vi "ELVIS III v1.0 Shutdown PWM.vi"(8 "error in (no error)":errorcluster, 10 "Channel":T1, 11 "myRIO Ref In":T2) -> (0 "error out":errorcluster, 3 "myRIO Ref Out":T2)   [LabVIEW 2021]
uses:
  <vilib>/myRIO/Common/Instrument Driver Framework/Utilities/typedefs/myRIO v1.0 Reference.ctl
  <vilib>/myRIO/Common/Instrument Driver Framework/Utilities/typedefs/Generic FPGA Reference.ctl
  <vilib>/myRIO/Common/Instrument Driver Framework/myRIO v1.0/PWM/typedefs/PWM Channels Enum.ctl
  <vilib>/myRIO/Common/Instrument Driver Framework/ELVIS III v1.0/PWM/typedefs/ELVIS III PWM Channels FPGA Reference.ctl
  <vilib>/rvi/errors/niLvFpgaAdjustHostInterfaceError.vi
  <vilib>/rvi/interface/nirviReadWriteControl/nirviReadWriteControl.xnode
  NiFpgaLv.dll
  <vilib>/rvi/interface/Simulation/niFpgaSimulationCallBeginRW.vi
panel:
  # "This VI turns off the specified PWM channel and zeroes out all of its registers."
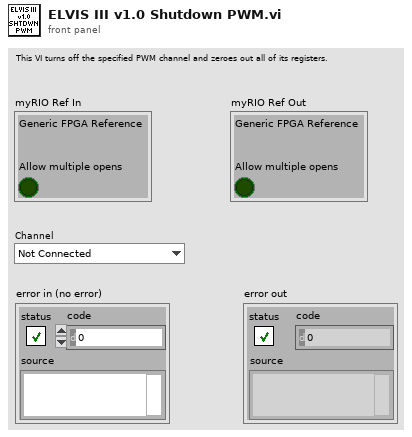
[diagram p1: front panel]
types:
  T1 = typedef "PWM Channels Enum.ctl" = enum16{"Not Connected", "C/PWM0", "C/PWM1", "A/PWM0", "A/PWM1", "A/PWM2", "A/PWM3", "A/PWM4", "A/PWM5", "A/PWM6", "A/PWM7", "A/PWM8", "A/PWM9", "A/PWM10", "A/PWM11", "A/PWM12", "A/PWM13", "A/PWM14", "A/PWM15", "A/PWM16", "A/PWM17", "A/PWM18", "A/PWM19", "B/PWM0", "B/PWM1", "B/PWM2", "B/PWM3", "B/PWM4", "B/PWM5", "B/PWM6", "B/PWM7", "B/PWM8", "B/PWM9", "B/PWM10", "B/PWM11", "B/PWM12", "B/PWM13", "B/PWM14", "B/PWM15", "B/PWM16", "B/PWM17", "B/PWM18", "B/PWM19", "PWM/PWM0", "PWM/PWM1", "PWM/PWM2", "PWM/PWM3", "PWM/PWM4", "PWM/PWM5", "PWM/PWM6", "PWM/PWM7", "PWM/PWM8", "PWM/PWM9"}
  T2 = typedef "myRIO v1.0 Reference.ctl" = cluster{"Generic FPGA Reference":T3, "Allow multiple opens":bool}
  T3 = typedef "Generic FPGA Reference.ctl" = refnum<k20>
  T4 = typedef "ELVIS III PWM Channels FPGA Reference.ctl" = refnum<k20>
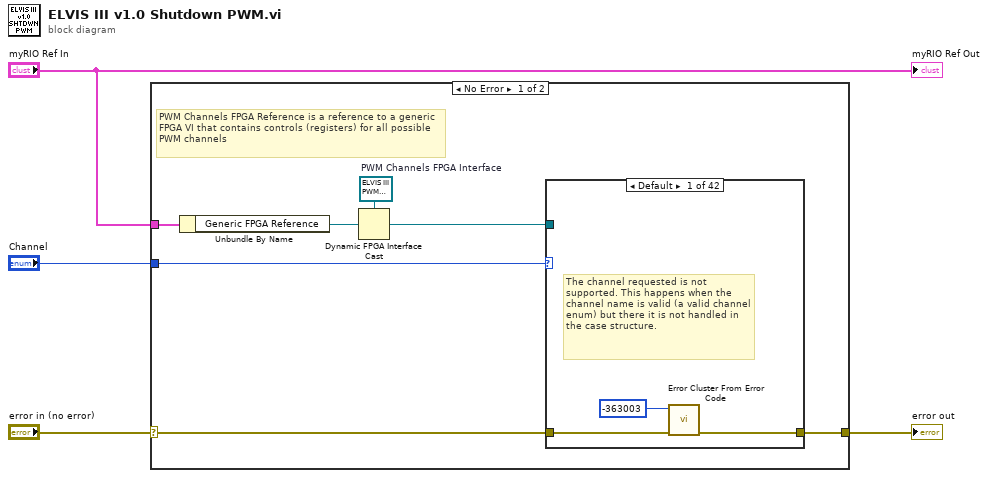
[diagram p0: block diagram]
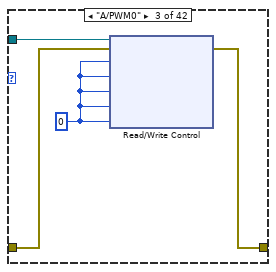
[diagram p3: hidden frame]
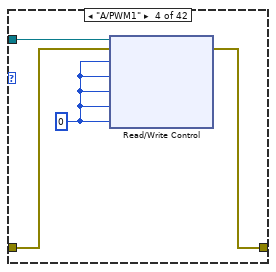
[diagram p4: hidden frame]
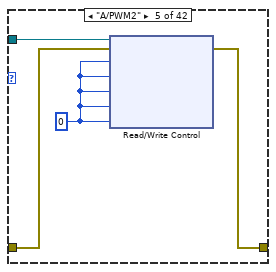
[diagram p5: hidden frame]
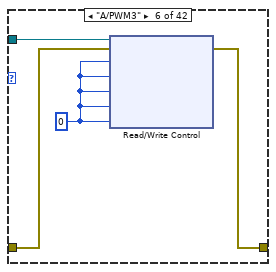
[diagram p6: hidden frame]
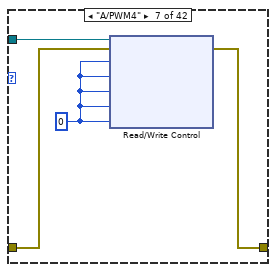
[diagram p7: hidden frame]
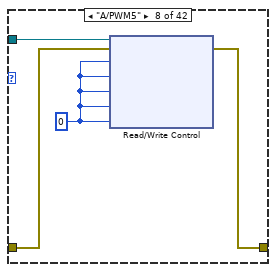
[diagram p8: hidden frame]
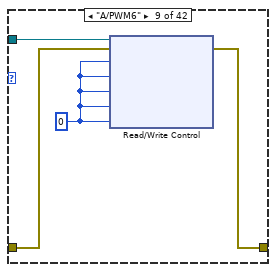
[diagram p9: hidden frame]
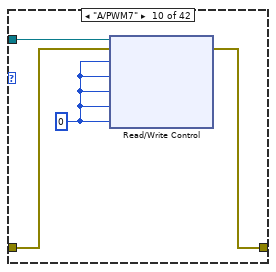
[diagram p10: hidden frame]
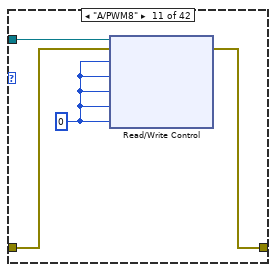
[diagram p11: hidden frame]
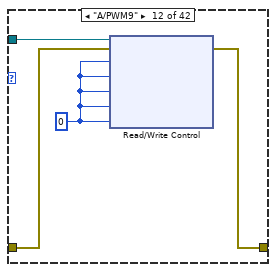
[diagram p12: hidden frame]
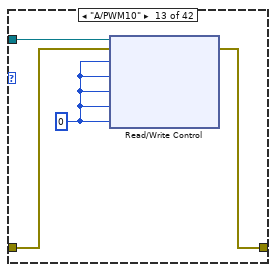
[diagram p13: hidden frame]
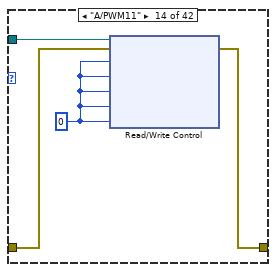
[diagram p14: hidden frame]
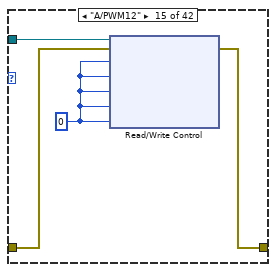
[diagram p15: hidden frame]
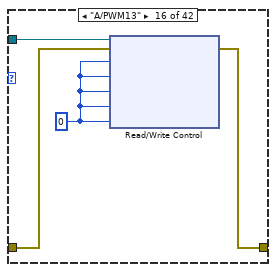
[diagram p16: hidden frame]
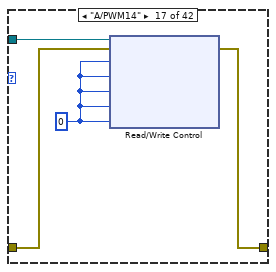
[diagram p17: hidden frame]
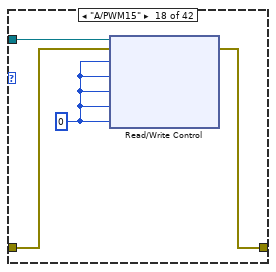
[diagram p18: hidden frame]
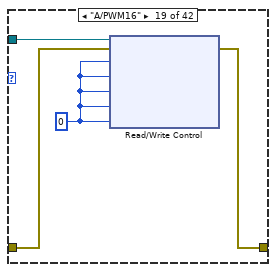
[diagram p19: hidden frame]
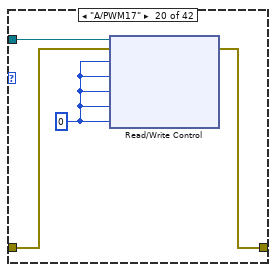
[diagram p20: hidden frame]
diagram:
  n1 = case shown="No Error" "error in (no error)" {
    selector: "error in (no error)" -> [w6 w176]
    tunnel: "myRIO Ref In" -> [w9 _]
    tunnel: [w8 w176] -> w3
    tunnel: "Channel" -> [w7 _]
    frame No Error {
      w11 = T4 refnum  # PWM Channels FPGA Interface
      # "PWM Channels FPGA Reference is a reference to a generic FPGA VI that contains controls (registers) for all possible PWM channels"
      n2 = Unbundle By Name(w9) -> ("Generic FPGA Reference"=w5:T3)
      n3 = Dynamic FPGA Interface Cast(Session In=w11, Type=w5) -> (Session Out=w10:T4)
      n4 = case shown="Default" w7 {
        tunnel: w6 -> [w12 w15 w17 w21 w25 w29 w33 w37 w41 w45 w49 w53 w57 w61 w65 w69 w73 w77 w81 w85 w89 w93 w97 w101 w105 w109 w113 w117 w121 w125 w129 w133 w137 w141 w145 w149 w153 w157 w161 w165 w169 w173]
        tunnel: [w13 w15 w16 w20 w24 w28 w32 w36 w40 w44 w48 w52 w56 w60 w64 w68 w72 w76 w80 w84 w88 w92 w96 w100 w104 w108 w112 w116 w120 w124 w128 w132 w136 w140 w144 w148 w152 w156 w160 w164 w168 w172] -> w8
        tunnel: w10 -> [_ _ w18 w22 w26 w30 w34 w38 w42 w46 w50 w54 w58 w62 w66 w70 w74 w78 w82 w86 w90 w94 w98 w102 w106 w110 w114 w118 w122 w126 w130 w134 w138 w142 w146 w150 w154 w158 w162 w166 w170 w174]
        frame Default {
          # "The channel requested is not supported. This happens when the channel name is valid (a valid channel enum) but there it is not handled in the case structure."
          n5 = call <vilib>:"Error Cluster From Error Code.vi"("error in (no error)"=w12, "error code (0)"=-363003) -> ("error out"=w13:errorcluster)  [unwired: 7 in]
        }
        frame "Not Connected" {
        }
        frame "A/PWM0" {
          w19 = u16 0 ("PWM.C_0.MAX")
          n6 = xnode "Read/Write Control"("FPGA VI Reference In"=w18, "error in"=w17, "PWM.A_0.CS"=w19, "PWM.A_0.CNFG"=w19, "PWM.A_0.CNTR"=w19, "PWM.A_0.CMP"=w19, "PWM.A_0.MAX"=w19) -> ("error out"=w16:errorcluster)  [unwired: 1 out]
        }
        frame "A/PWM1" {
          w23 = u16 0 ("PWM.C_0.MAX")
          n7 = xnode "Read/Write Control"("FPGA VI Reference In"=w22, "error in"=w21, "PWM.A_1.CS"=w23, "PWM.A_1.CNFG"=w23, "PWM.A_1.CNTR"=w23, "PWM.A_1.CMP"=w23, "PWM.A_1.MAX"=w23) -> ("error out"=w20:errorcluster)  [unwired: 1 out]
        }
        frame "A/PWM2" {
          w27 = u16 0 ("PWM.C_0.MAX")
          n8 = xnode "Read/Write Control"("FPGA VI Reference In"=w26, "error in"=w25, "PWM.A_2.CS"=w27, "PWM.A_2.CNFG"=w27, "PWM.A_2.CNTR"=w27, "PWM.A_2.CMP"=w27, "PWM.A_2.MAX"=w27) -> ("error out"=w24:errorcluster)  [unwired: 1 out]
        }
        frame "A/PWM3" {
          w31 = u16 0 ("PWM.C_0.MAX")
          n9 = xnode "Read/Write Control"("FPGA VI Reference In"=w30, "error in"=w29, "PWM.A_3.CS"=w31, "PWM.A_3.CNFG"=w31, "PWM.A_3.CNTR"=w31, "PWM.A_3.CMP"=w31, "PWM.A_3.MAX"=w31) -> ("error out"=w28:errorcluster)  [unwired: 1 out]
        }
        frame "A/PWM4" {
          w35 = u16 0 ("PWM.C_0.MAX")
          n10 = xnode "Read/Write Control"("FPGA VI Reference In"=w34, "error in"=w33, "PWM.A_4.CS"=w35, "PWM.A_4.CNFG"=w35, "PWM.A_4.CNTR"=w35, "PWM.A_4.CMP"=w35, "PWM.A_4.MAX"=w35) -> ("error out"=w32:errorcluster)  [unwired: 1 out]
        }
        frame "A/PWM5" {
          w39 = u16 0 ("PWM.C_0.MAX")
          n11 = xnode "Read/Write Control"("FPGA VI Reference In"=w38, "error in"=w37, "PWM.A_5.CS"=w39, "PWM.A_5.CNFG"=w39, "PWM.A_5.CNTR"=w39, "PWM.A_5.CMP"=w39, "PWM.A_5.MAX"=w39) -> ("error out"=w36:errorcluster)  [unwired: 1 out]
        }
        frame "A/PWM6" {
          w43 = u16 0 ("PWM.C_0.MAX")
          n12 = xnode "Read/Write Control"("FPGA VI Reference In"=w42, "error in"=w41, "PWM.A_6.CS"=w43, "PWM.A_6.CNFG"=w43, "PWM.A_6.CNTR"=w43, "PWM.A_6.CMP"=w43, "PWM.A_6.MAX"=w43) -> ("error out"=w40:errorcluster)  [unwired: 1 out]
        }
        frame "A/PWM7" {
          w47 = u16 0 ("PWM.C_0.MAX")
          n13 = xnode "Read/Write Control"("FPGA VI Reference In"=w46, "error in"=w45, "PWM.A_7.CS"=w47, "PWM.A_7.CNFG"=w47, "PWM.A_7.CNTR"=w47, "PWM.A_7.CMP"=w47, "PWM.A_7.MAX"=w47) -> ("error out"=w44:errorcluster)  [unwired: 1 out]
        }
        frame "A/PWM8" {
          w51 = u16 0 ("PWM.C_0.MAX")
          n14 = xnode "Read/Write Control"("FPGA VI Reference In"=w50, "error in"=w49, "PWM.A_8.CS"=w51, "PWM.A_8.CNFG"=w51, "PWM.A_8.CNTR"=w51, "PWM.A_8.CMP"=w51, "PWM.A_8.MAX"=w51) -> ("error out"=w48:errorcluster)  [unwired: 1 out]
        }
        frame "A/PWM9" {
          w55 = u16 0 ("PWM.C_0.MAX")
          n15 = xnode "Read/Write Control"("FPGA VI Reference In"=w54, "error in"=w53, "PWM.A_9.CS"=w55, "PWM.A_9.CNFG"=w55, "PWM.A_9.CNTR"=w55, "PWM.A_9.CMP"=w55, "PWM.A_9.MAX"=w55) -> ("error out"=w52:errorcluster)  [unwired: 1 out]
        }
        frame "A/PWM10" {
          w59 = u16 0 ("PWM.C_0.MAX")
          n16 = xnode "Read/Write Control"("FPGA VI Reference In"=w58, "error in"=w57, "PWM.A_10.CS"=w59, "PWM.A_10.CNFG"=w59, "PWM.A_10.CNTR"=w59, "PWM.A_10.CMP"=w59, "PWM.A_10.MAX"=w59) -> ("error out"=w56:errorcluster)  [unwired: 1 out]
        }
        frame "A/PWM11" {
          w63 = u16 0 ("PWM.C_0.MAX")
          n17 = xnode "Read/Write Control"("FPGA VI Reference In"=w62, "error in"=w61, "PWM.A_11.CS"=w63, "PWM.A_11.CNFG"=w63, "PWM.A_11.CNTR"=w63, "PWM.A_11.CMP"=w63, "PWM.A_11.MAX"=w63) -> ("error out"=w60:errorcluster)  [unwired: 1 out]
        }
        frame "A/PWM12" {
          w67 = u16 0 ("PWM.C_0.MAX")
          n18 = xnode "Read/Write Control"("FPGA VI Reference In"=w66, "error in"=w65, "PWM.A_12.CS"=w67, "PWM.A_12.CNFG"=w67, "PWM.A_12.CNTR"=w67, "PWM.A_12.CMP"=w67, "PWM.A_12.MAX"=w67) -> ("error out"=w64:errorcluster)  [unwired: 1 out]
        }
        frame "A/PWM13" {
          w71 = u16 0 ("PWM.C_0.MAX")
          n19 = xnode "Read/Write Control"("FPGA VI Reference In"=w70, "error in"=w69, "PWM.A_13.CS"=w71, "PWM.A_13.CNFG"=w71, "PWM.A_13.CNTR"=w71, "PWM.A_13.CMP"=w71, "PWM.A_13.MAX"=w71) -> ("error out"=w68:errorcluster)  [unwired: 1 out]
        }
        frame "A/PWM14" {
          w75 = u16 0 ("PWM.C_0.MAX")
          n20 = xnode "Read/Write Control"("FPGA VI Reference In"=w74, "error in"=w73, "PWM.A_14.CS"=w75, "PWM.A_14.CNFG"=w75, "PWM.A_14.CNTR"=w75, "PWM.A_14.CMP"=w75, "PWM.A_14.MAX"=w75) -> ("error out"=w72:errorcluster)  [unwired: 1 out]
        }
        frame "A/PWM15" {
          w79 = u16 0 ("PWM.C_0.MAX")
          n21 = xnode "Read/Write Control"("FPGA VI Reference In"=w78, "error in"=w77, "PWM.A_15.CS"=w79, "PWM.A_15.CNFG"=w79, "PWM.A_15.CNTR"=w79, "PWM.A_15.CMP"=w79, "PWM.A_15.MAX"=w79) -> ("error out"=w76:errorcluster)  [unwired: 1 out]
        }
        frame "A/PWM16" {
          w83 = u16 0 ("PWM.C_0.MAX")
          n22 = xnode "Read/Write Control"("FPGA VI Reference In"=w82, "error in"=w81, "PWM.A_16.CS"=w83, "PWM.A_16.CNFG"=w83, "PWM.A_16.CNTR"=w83, "PWM.A_16.CMP"=w83, "PWM.A_16.MAX"=w83) -> ("error out"=w80:errorcluster)  [unwired: 1 out]
        }
        frame "A/PWM17" {
          w87 = u16 0 ("PWM.C_0.MAX")
          n23 = xnode "Read/Write Control"("FPGA VI Reference In"=w86, "error in"=w85, "PWM.A_17.CS"=w87, "PWM.A_17.CNFG"=w87, "PWM.A_17.CNTR"=w87, "PWM.A_17.CMP"=w87, "PWM.A_17.MAX"=w87) -> ("error out"=w84:errorcluster)  [unwired: 1 out]
        }
        frame "A/PWM18" {
          w91 = u16 0 ("PWM.C_0.MAX")
          n24 = xnode "Read/Write Control"("FPGA VI Reference In"=w90, "error in"=w89, "PWM.A_18.CS"=w91, "PWM.A_18.CNFG"=w91, "PWM.A_18.CNTR"=w91, "PWM.A_18.CMP"=w91, "PWM.A_18.MAX"=w91) -> ("error out"=w88:errorcluster)  [unwired: 1 out]
        }
        frame "A/PWM19" {
          w95 = u16 0 ("PWM.C_0.MAX")
          n25 = xnode "Read/Write Control"("FPGA VI Reference In"=w94, "error in"=w93, "PWM.A_19.CS"=w95, "PWM.A_19.CNFG"=w95, "PWM.A_19.CNTR"=w95, "PWM.A_19.CMP"=w95, "PWM.A_19.MAX"=w95) -> ("error out"=w92:errorcluster)  [unwired: 1 out]
        }
        frame "B/PWM0" {
          w99 = u16 0 ("PWM.C_0.MAX")
          n26 = xnode "Read/Write Control"("FPGA VI Reference In"=w98, "error in"=w97, "PWM.B_0.CS"=w99, "PWM.B_0.CNFG"=w99, "PWM.B_0.CNTR"=w99, "PWM.B_0.CMP"=w99, "PWM.B_0.MAX"=w99) -> ("error out"=w96:errorcluster)  [unwired: 1 out]
        }
        frame "B/PWM1" {
          w103 = u16 0 ("PWM.C_0.MAX")
          n27 = xnode "Read/Write Control"("FPGA VI Reference In"=w102, "error in"=w101, "PWM.B_1.CS"=w103, "PWM.B_1.CNFG"=w103, "PWM.B_1.CNTR"=w103, "PWM.B_1.CMP"=w103, "PWM.B_1.MAX"=w103) -> ("error out"=w100:errorcluster)  [unwired: 1 out]
        }
        frame "B/PWM2" {
          w107 = u16 0 ("PWM.C_0.MAX")
          n28 = xnode "Read/Write Control"("FPGA VI Reference In"=w106, "error in"=w105, "PWM.B_2.CS"=w107, "PWM.B_2.CNFG"=w107, "PWM.B_2.CNTR"=w107, "PWM.B_2.CMP"=w107, "PWM.B_2.MAX"=w107) -> ("error out"=w104:errorcluster)  [unwired: 1 out]
        }
        frame "B/PWM3" {
          w111 = u16 0 ("PWM.C_0.MAX")
          n29 = xnode "Read/Write Control"("FPGA VI Reference In"=w110, "error in"=w109, "PWM.B_3.CS"=w111, "PWM.B_3.CNFG"=w111, "PWM.B_3.CNTR"=w111, "PWM.B_3.CMP"=w111, "PWM.B_3.MAX"=w111) -> ("error out"=w108:errorcluster)  [unwired: 1 out]
        }
        frame "B/PWM4" {
          w115 = u16 0 ("PWM.C_0.MAX")
          n30 = xnode "Read/Write Control"("FPGA VI Reference In"=w114, "error in"=w113, "PWM.B_4.CS"=w115, "PWM.B_4.CNFG"=w115, "PWM.B_4.CNTR"=w115, "PWM.B_4.CMP"=w115, "PWM.B_4.MAX"=w115) -> ("error out"=w112:errorcluster)  [unwired: 1 out]
        }
        frame "B/PWM5" {
          w119 = u16 0 ("PWM.C_0.MAX")
          n31 = xnode "Read/Write Control"("FPGA VI Reference In"=w118, "error in"=w117, "PWM.B_5.CS"=w119, "PWM.B_5.CNFG"=w119, "PWM.B_5.CNTR"=w119, "PWM.B_5.CMP"=w119, "PWM.B_5.MAX"=w119) -> ("error out"=w116:errorcluster)  [unwired: 1 out]
        }
        frame "B/PWM6" {
          w123 = u16 0 ("PWM.C_0.MAX")
          n32 = xnode "Read/Write Control"("FPGA VI Reference In"=w122, "error in"=w121, "PWM.B_6.CS"=w123, "PWM.B_6.CNFG"=w123, "PWM.B_6.CNTR"=w123, "PWM.B_6.CMP"=w123, "PWM.B_6.MAX"=w123) -> ("error out"=w120:errorcluster)  [unwired: 1 out]
        }
        frame "B/PWM7" {
          w127 = u16 0 ("PWM.C_0.MAX")
          n33 = xnode "Read/Write Control"("FPGA VI Reference In"=w126, "error in"=w125, "PWM.B_7.CS"=w127, "PWM.B_7.CNFG"=w127, "PWM.B_7.CNTR"=w127, "PWM.B_7.CMP"=w127, "PWM.B_7.MAX"=w127) -> ("error out"=w124:errorcluster)  [unwired: 1 out]
        }
        frame "B/PWM8" {
          w131 = u16 0 ("PWM.C_0.MAX")
          n34 = xnode "Read/Write Control"("FPGA VI Reference In"=w130, "error in"=w129, "PWM.B_8.CS"=w131, "PWM.B_8.CNFG"=w131, "PWM.B_8.CNTR"=w131, "PWM.B_8.CMP"=w131, "PWM.B_8.MAX"=w131) -> ("error out"=w128:errorcluster)  [unwired: 1 out]
        }
        frame "B/PWM9" {
          w135 = u16 0 ("PWM.C_0.MAX")
          n35 = xnode "Read/Write Control"("FPGA VI Reference In"=w134, "error in"=w133, "PWM.B_9.CS"=w135, "PWM.B_9.CNFG"=w135, "PWM.B_9.CNTR"=w135, "PWM.B_9.CMP"=w135, "PWM.B_9.MAX"=w135) -> ("error out"=w132:errorcluster)  [unwired: 1 out]
        }
        frame "B/PWM10" {
          w139 = u16 0 ("PWM.C_0.MAX")
          n36 = xnode "Read/Write Control"("FPGA VI Reference In"=w138, "error in"=w137, "PWM.B_10.CS"=w139, "PWM.B_10.CNFG"=w139, "PWM.B_10.CNTR"=w139, "PWM.B_10.CMP"=w139, "PWM.B_10.MAX"=w139) -> ("error out"=w136:errorcluster)  [unwired: 1 out]
        }
        frame "B/PWM11" {
          w143 = u16 0 ("PWM.C_0.MAX")
          n37 = xnode "Read/Write Control"("FPGA VI Reference In"=w142, "error in"=w141, "PWM.B_11.CS"=w143, "PWM.B_11.CNFG"=w143, "PWM.B_11.CNTR"=w143, "PWM.B_11.CMP"=w143, "PWM.B_11.MAX"=w143) -> ("error out"=w140:errorcluster)  [unwired: 1 out]
        }
        frame "B/PWM12" {
          w147 = u16 0 ("PWM.C_0.MAX")
          n38 = xnode "Read/Write Control"("FPGA VI Reference In"=w146, "error in"=w145, "PWM.B_12.CS"=w147, "PWM.B_12.CNFG"=w147, "PWM.B_12.CNTR"=w147, "PWM.B_12.CMP"=w147, "PWM.B_12.MAX"=w147) -> ("error out"=w144:errorcluster)  [unwired: 1 out]
        }
        frame "B/PWM13" {
          w151 = u16 0 ("PWM.C_0.MAX")
          n39 = xnode "Read/Write Control"("FPGA VI Reference In"=w150, "error in"=w149, "PWM.B_13.CS"=w151, "PWM.B_13.CNFG"=w151, "PWM.B_13.CNTR"=w151, "PWM.B_13.CMP"=w151, "PWM.B_13.MAX"=w151) -> ("error out"=w148:errorcluster)  [unwired: 1 out]
        }
        frame "B/PWM14" {
          w155 = u16 0 ("PWM.C_0.MAX")
          n40 = xnode "Read/Write Control"("FPGA VI Reference In"=w154, "error in"=w153, "PWM.B_14.CS"=w155, "PWM.B_14.CNFG"=w155, "PWM.B_14.CNTR"=w155, "PWM.B_14.CMP"=w155, "PWM.B_14.MAX"=w155) -> ("error out"=w152:errorcluster)  [unwired: 1 out]
        }
        frame "B/PWM15" {
          w159 = u16 0 ("PWM.C_0.MAX")
          n41 = xnode "Read/Write Control"("FPGA VI Reference In"=w158, "error in"=w157, "PWM.B_15.CS"=w159, "PWM.B_15.CNFG"=w159, "PWM.B_15.CNTR"=w159, "PWM.B_15.CMP"=w159, "PWM.B_15.MAX"=w159) -> ("error out"=w156:errorcluster)  [unwired: 1 out]
        }
        frame "B/PWM16" {
          w163 = u16 0 ("PWM.C_0.MAX")
          n42 = xnode "Read/Write Control"("FPGA VI Reference In"=w162, "error in"=w161, "PWM.B_16.CS"=w163, "PWM.B_16.CNFG"=w163, "PWM.B_16.CNTR"=w163, "PWM.B_16.CMP"=w163, "PWM.B_16.MAX"=w163) -> ("error out"=w160:errorcluster)  [unwired: 1 out]
        }
        frame "B/PWM17" {
          w167 = u16 0 ("PWM.C_0.MAX")
          n43 = xnode "Read/Write Control"("FPGA VI Reference In"=w166, "error in"=w165, "PWM.B_17.CS"=w167, "PWM.B_17.CNFG"=w167, "PWM.B_17.CNTR"=w167, "PWM.B_17.CMP"=w167, "PWM.B_17.MAX"=w167) -> ("error out"=w164:errorcluster)  [unwired: 1 out]
        }
        frame "B/PWM18" {
          w171 = u16 0 ("PWM.C_0.MAX")
          n44 = xnode "Read/Write Control"("FPGA VI Reference In"=w170, "error in"=w169, "PWM.B_18.CS"=w171, "PWM.B_18.CNFG"=w171, "PWM.B_18.CNTR"=w171, "PWM.B_18.CMP"=w171, "PWM.B_18.MAX"=w171) -> ("error out"=w168:errorcluster)  [unwired: 1 out]
        }
        frame "B/PWM19" {
          w175 = u16 0 ("PWM.C_0.MAX")
          n45 = xnode "Read/Write Control"("FPGA VI Reference In"=w174, "error in"=w173, "PWM.B_19.CS"=w175, "PWM.B_19.CNFG"=w175, "PWM.B_19.CNTR"=w175, "PWM.B_19.CMP"=w175, "PWM.B_19.MAX"=w175) -> ("error out"=w172:errorcluster)  [unwired: 1 out]
        }
      }
    }
    frame Error {
      # "Nothing to do since there was an incoming error."
    }
  }
  "error out" <- w3
  "myRIO Ref Out" <- "myRIO Ref In"
